vi "Control Scan.vi"(8 "error in (no error)":errorcluster, 9 "Internal Scanner Control Channel ((@ 1:10))":string="(@ 1:10)", 10 "Scanner Control (0: Open All)":i32(ring) items=["Open All", "Open List", "Close List"], 11 "VISA resource name":refnum<visa-resource-name>) -> (0 "error out":errorcluster, 3 "VISA resource name out":refnum<visa-resource-name>)   [LabVIEW 2019, in "Keithley 6517.lvlib"]
doc: "Opens or closes the specified channel.\n\nNote:\nRequires a separate scanner card. According to the manual 6521 or 6522, 7001 and 7002 can be used with this model. If the scanner card is not used the error -241, \"Hardware missing\" will be generated.\n\nThis VI is <B>NOT</B> compatible with model <B>6514</B>."
uses:
  Keithley 6517.lvlib
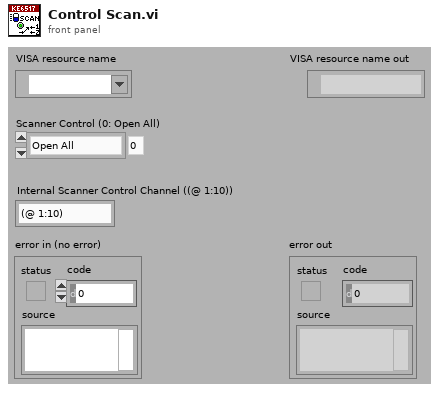
[diagram p1: front panel]
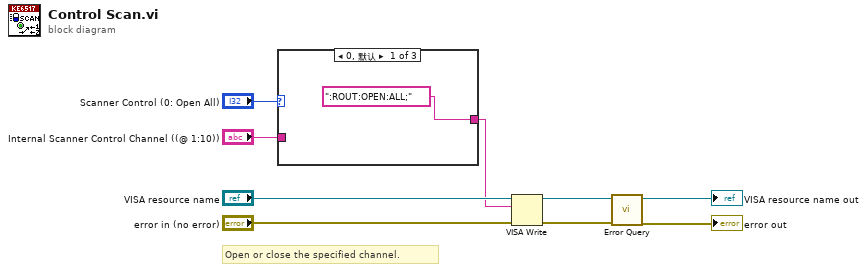
[diagram p0: block diagram]
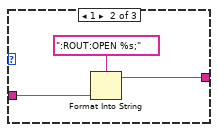
[diagram p2: hidden frame]
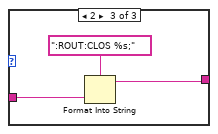
[diagram p3: hidden frame]
diagram:
  # "Open or close the specified channel."
  n1 = case shown="0, 默认" "Scanner Control (0: Open All)" {
    tunnel: [":ROUT:OPEN:ALL;" w11 w14] -> w2
    tunnel: "Internal Scanner Control Channel ((@ 1:10))" -> [_ w12 w15]
    frame 0, Default {
    }
    frame 1 {
      n2 = Format Into String(format string=":ROUT:OPEN %s;", w12) -> (resulting string=w11:string)  [unwired: 2 in, 1 out]
    }
    frame 2 {
      n3 = Format Into String(format string=":ROUT:CLOS %s;", w15) -> (resulting string=w14:string)  [unwired: 2 in, 1 out]
    }
  }
  n4 = VISA Write(VISA resource name="VISA resource name", write buffer=w2, error in (no error)="error in (no error)") -> (VISA resource name out=w7:refnum<visa-resource-name>, error out=w6:errorcluster)  [unwired: 1 out]
  n5 = call "Error Query.vi"("error in (no error)"=w6, "VISA resource name"=w7) -> ("error out"=→"error out":errorcluster, "VISA resource name out"=→"VISA resource name out":refnum<visa-resource-name>)  [unwired: 6 in, 2 out]
